vi "IR_PARA_00.vi"(8 "Parâmetros":T3={"Verde Min "=0.0, "Verde  MAX"=4.0, "Vemelho Max"=0, "Azul Max"=0, "Amarelo Max"=0, "Chão Max"=0.0, "Branco Max EV3 Cor"=0.0, "Branco Min EV3 Cor"=0.0, "Preto Max EV3 Cor"=0.0, "Preto Min EV3 Cor"=0.0, "Tubo CM Max"=0.0, "Tubo CM Min"=0.0, "Dist Proxima"=0.0, "Graus Emp"=0, "Graus Aprox"=0, "Graus Afast"=0, "180dg"=170.0, "90dg"=80.0, "Vemelho Min"=0, "Azul  Min"=0, "Amarelo Min"=0, "Chão Min"=0.0}, 11 "NXT/EV3":T2) -> (3 "NXT/EV3 2":T2)   [LabVIEW 2016]
uses:
  <vilib>/NXT/LegoClasses/BrickReference/BrickReference.lvclass
  <vilib>/NXT/Subs/LVHSConnector.ctl
  <vilib>/NXT/Block Support/NXT_OutputPort.ctl
  <vilib>/NXT/Dual Mode Library/Sensors/EV3_Color_Reflect.vi
  <vilib>/NXT/NXTIO Xnodes/NXTIONodeSubVIs/NXTStopMotors.vi
  <vilib>/NXT/NXTIO Xnodes/AddressXNode/NXTIOAddress.xnode
  <vilib>/NXT/NXTIO Xnodes/NXTIOXNode/NXTIO.xnode
panel:
  out "x+1":i32
  in  "Numeric":i32
  in  "Parâmetros\n CHÃO":T1={"Branco HiTechnic"=17, "Preto HiTechnic"=0, "Verde HiTechnic"=6, "Vemelho HiTechnic"=0, "Azul HiTechnic"=0, "Amarelo HiTechnic"=0, "Chão EV3 Cor"=0.0, "Branco Max EV3 Cor"=0.0, "Branco Min EV3 Cor"=0.0, "Preto Max EV3 Cor"=0.0, "Preto Min EV3 Cor"=0.0, "Tubo CM Max"=0.0, "Tubo CM Min"=0.0, "Dist Proxima"=0.0, "Graus Emp"=0, "Graus Aprox"=0, "Graus Afast"=0, "180dg"=0.0, "90dg"=0.0}
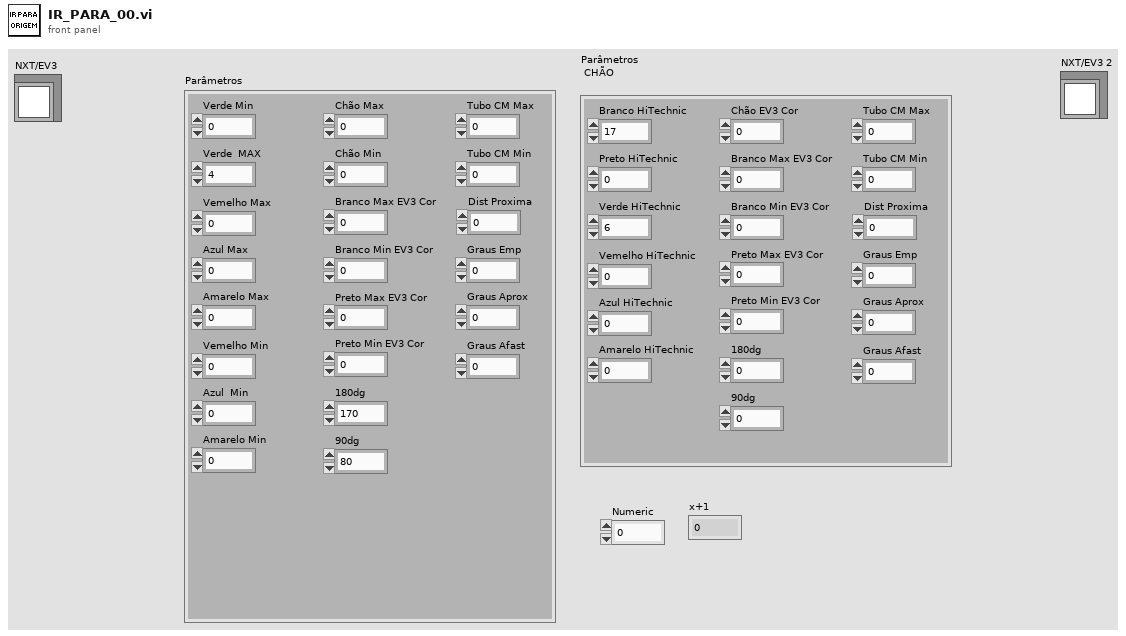
[diagram p1: front panel]
types:
  T1 = cluster{"Branco HiTechnic":i32, "Preto HiTechnic":i32, "Verde HiTechnic":i32, "Vemelho HiTechnic":i32, "Azul HiTechnic":i32, "Amarelo HiTechnic":i32, "Chão EV3 Cor":sgl, "Branco Max EV3 Cor":sgl, "Branco Min EV3 Cor":sgl, "Preto Max EV3 Cor":sgl, "Preto Min EV3 Cor":sgl, "Tubo CM Max":sgl, "Tubo CM Min":sgl, "Dist Proxima":dbl, "Graus Emp":i32, "Graus Aprox":i32, "Graus Afast":i32, "180dg":sgl, "90dg":sgl}
  T2 = typedef "LVHSConnector.ctl" = refnum<class "BrickReference.lvclass">
  T3 = cluster{"Verde Min ":dbl, "Verde  MAX":dbl, "Vemelho Max":i32, "Azul Max":i32, "Amarelo Max":i32, "Chão Max":sgl, "Branco Max EV3 Cor":sgl, "Branco Min EV3 Cor":sgl, "Preto Max EV3 Cor":sgl, "Preto Min EV3 Cor":sgl, "Tubo CM Max":sgl, "Tubo CM Min":sgl, "Dist Proxima":dbl, "Graus Emp":i32, "Graus Aprox":i32, "Graus Afast":i32, "180dg":sgl, "90dg":sgl, "Vemelho Min":i32, "Azul  Min":i32, "Amarelo Min":i32, "Chão Min":sgl}
  T4 = typedef "NXT_OutputPort.ctl" = u8
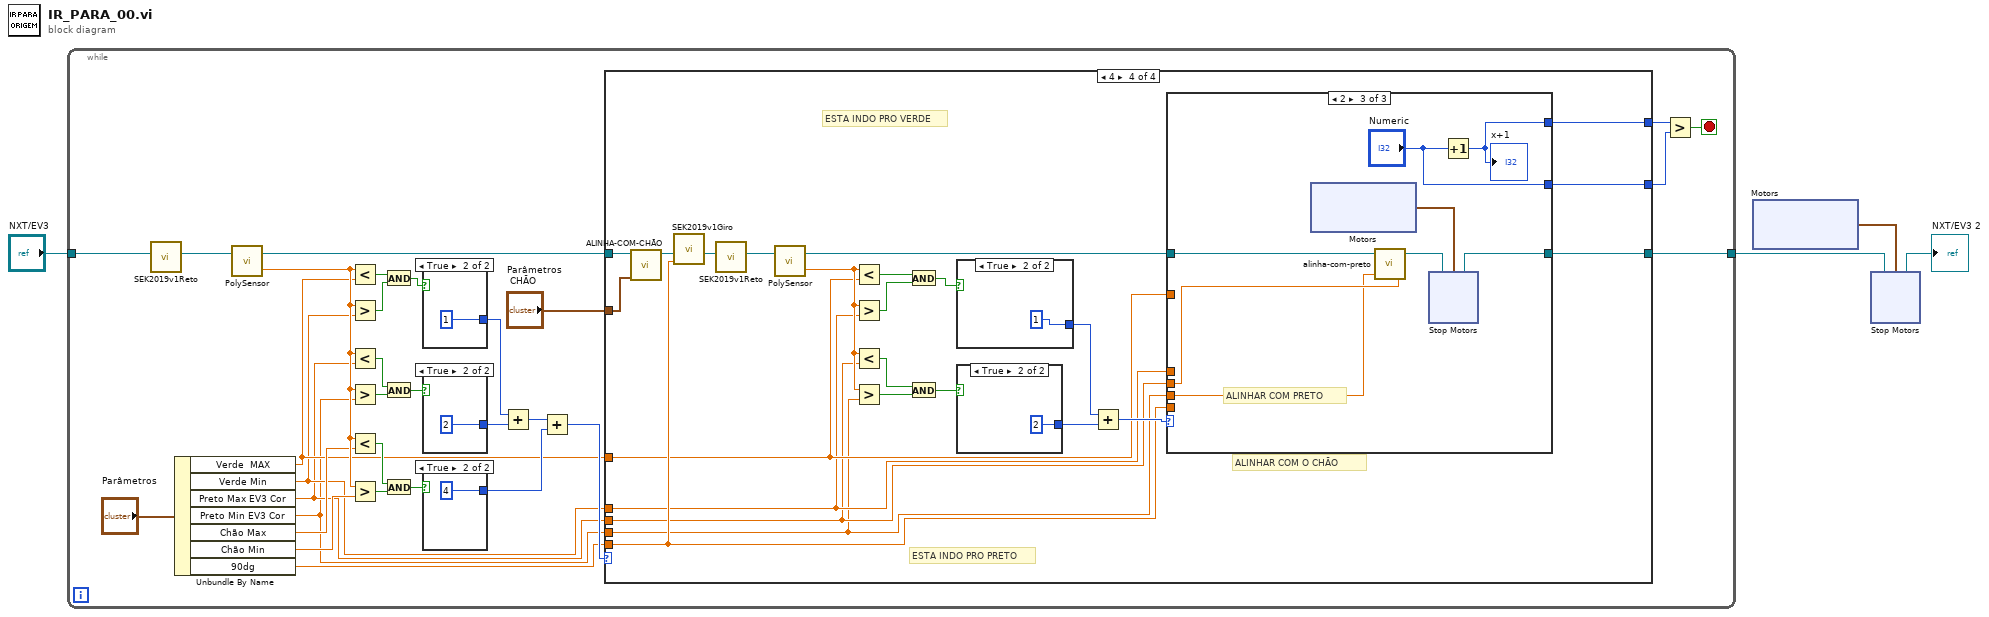
[diagram p0: block diagram]
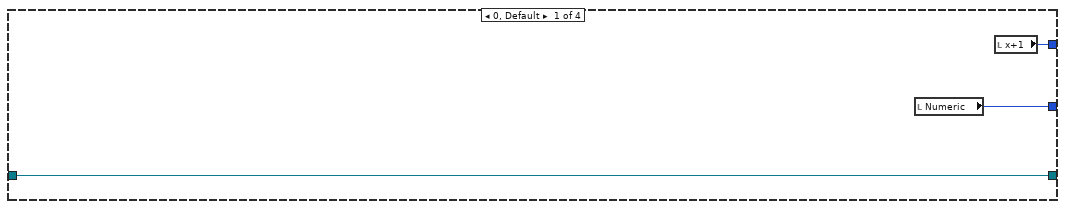
[diagram p2: hidden frame]
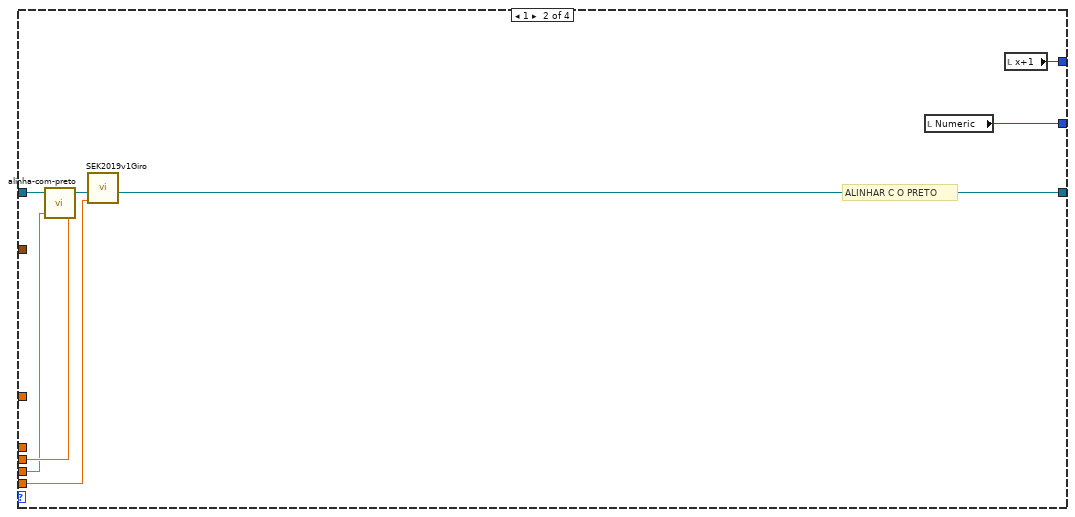
[diagram p3: hidden frame]
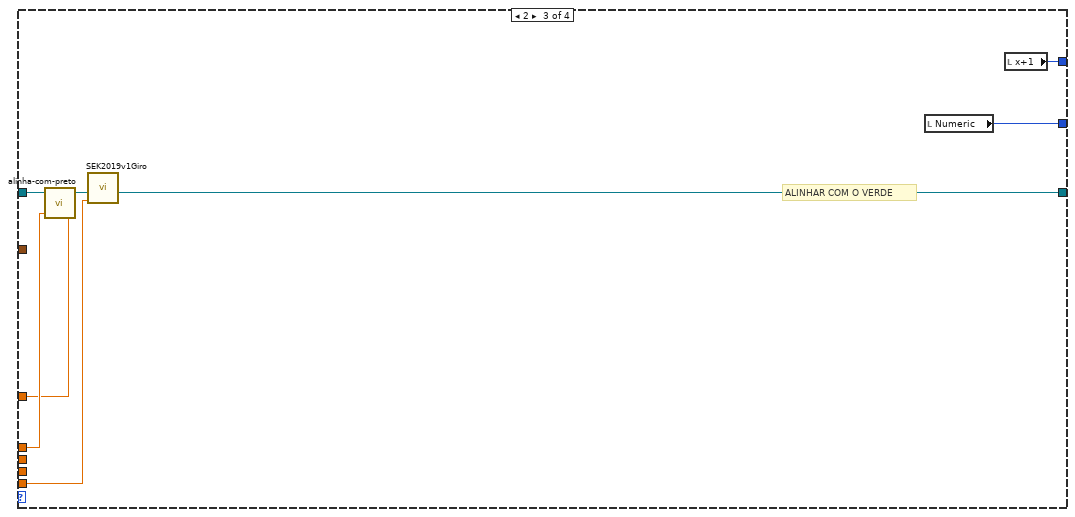
[diagram p4: hidden frame]
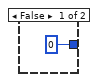
[diagram p5: hidden frame]
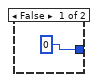
[diagram p6: hidden frame]
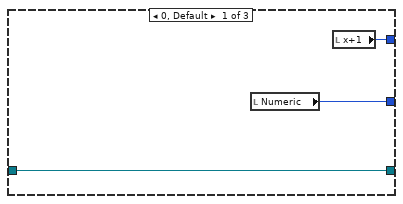
[diagram p7: hidden frame]
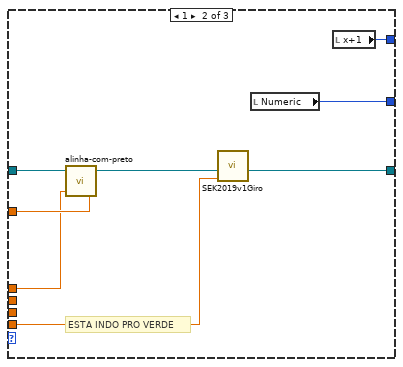
[diagram p8: hidden frame]
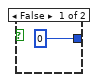
[diagram p9: hidden frame]
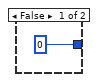
[diagram p10: hidden frame]
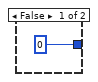
[diagram p11: hidden frame]
diagram:
  n1 = while {
    tunnel: "NXT/EV3" -> [w16]
    tunnel: [w9] -> w1
    stop <- w10 stop-if-true
    n2 = call "SEK2019v1Reto.vi"("NXT/EV3"=w16) -> ("NXT/EV3 2"=w15:T2)  [unwired: 10 in]
    n3 = Unbundle By Name("Parâmetros") -> ("Verde  MAX"=w8:dbl, "Verde Min"=w7:dbl, "Preto Max EV3 Cor"=w6:sgl, "Preto Min EV3 Cor"=w5:sgl, "Chão Max"=w28:sgl, "Chão Min"=w27:sgl, "90dg"=w14:sgl)
    n4 = call-poly <vilib>:"PolySensor.vi"("NXT/EV3"=w15) -> ("Scaled Value"=w29:sgl, "NXT/EV3"=w17:T2)  [unwired: 2 in]
    n5 = Less?(x=w29, y=w8) -> (x < y?=w21:bool)
    n6 = Greater?(x=w29, y=w7) -> (0:w22:bool)
    n7 = Less?(x=w29, y=w6) -> (x < y?=w24:bool)
    n8 = Greater?(x=w29, y=w5) -> (0:w23:bool)
    n9 = Less?(x=w29, y=w28) -> (x < y?=w26:bool)
    n10 = Greater?(x=w29, y=w27) -> (0:w25:bool)
    n11 = And(x=w21, y=w22) -> (x .and. y?=w20:bool)
    n12 = And(x=w24, y=w23) -> (x .and. y?=w19:bool)
    n13 = And(x=w26, y=w25) -> (x .and. y?=w18:bool)
    n14 = case shown="True" w20 {
      tunnel: [0 1] -> w34
      frame False {
      }
      frame True {
      }
    }
    n15 = case shown="True" w19 {
      tunnel: [0 2] -> w33
      frame False {
      }
      frame True {
      }
    }
    n16 = case shown="True" w18 {
      tunnel: [0 4] -> w32
      frame False {
      }
      frame True {
      }
    }
    n17 = Add(x=w34, y=w33) -> (x+y=w31:i32)
    n18 = Add(x=w31, y=w32) -> (x+y=w30:i32)
    n19 = case shown="4" w30 {
      tunnel: w8 -> [_ _ w53 w63]
      tunnel: w7 -> [_ _ w54 w62]
      tunnel: w6 -> [_ w46 _ w61]
      tunnel: w5 -> [_ w45 _ w60]
      tunnel: w17 -> [w38 w44 w52 w78]
      tunnel: [w38 w41 w50 w58] -> w9
      tunnel: w14 -> [_ w43 w49 w64]
      tunnel: "Parâmetros\n CHÃO" -> [_ _ _ w57]
      tunnel: [w37 w39 w48 w56] -> w12
      tunnel: [w36 w40 w47 w55] -> w11
      frame 0, Default {
        n20 = local read "Numeric"() -> (w37:i32)
        n21 = local read "x+1"() -> (w36:i32)
      }
      frame 1 {
        # "ALINHAR C O PRETO"
        n22 = call "alinha-com-preto.vi"("COR 2 Max EV3 Cor"=w46, "COR 2 Min EV3 Cor"=w45, "NXT/EV3"=w44) -> ("NXT/EV3 2"=w42:T2)  [unwired: 2 in]
        n23 = call "SEK2019v1Giro.vi"("ANGULO"=w43, "NXT/EV3"=w42) -> ("NXT/EV3 2"=w41:T2)  [unwired: 9 in]
        n24 = local read "Numeric"() -> (w39:i32)
        n25 = local read "x+1"() -> (w40:i32)
      }
      frame 2 {
        # "ALINHAR COM O VERDE"
        n26 = call "alinha-com-preto.vi"("COR 2 Max EV3 Cor"=w53, "COR 2 Min EV3 Cor"=w54, "NXT/EV3"=w52) -> ("NXT/EV3 2"=w51:T2)  [unwired: 2 in]
        n27 = call "SEK2019v1Giro.vi"("ANGULO"=w49, "NXT/EV3"=w51) -> ("NXT/EV3 2"=w50:T2)  [unwired: 9 in]
        n28 = local read "Numeric"() -> (w48:i32)
        n29 = local read "x+1"() -> (w47:i32)
      }
      frame 4 {
        # "ESTA INDO PRO VERDE"
        # "ESTA INDO PRO PRETO"
        # "ALINHAR COM O CHÃO"
        n30 = call "ALINHA-COM-CHÃO.vi"("Parâmetros"=w57, "NXT/EV3"=w78) -> ("NXT/EV3 2"=w77:T2)  [unwired: 9 in]
        n31 = call "SEK2019v1Giro.vi"("ANGULO"=w64, "NXT/EV3"=w77) -> ("NXT/EV3 2"=w76:T2)  [unwired: 9 in]
        n32 = call "SEK2019v1Reto.vi"("NXT/EV3"=w76) -> ("NXT/EV3 2"=w70:T2)  [unwired: 10 in]
        n33 = call-poly <vilib>:"PolySensor.vi"("NXT/EV3"=w70) -> ("Scaled Value"=w71:sgl, "NXT/EV3"=w59:T2)  [unwired: 2 in]
        n34 = Less?(x=w71, y=w63) -> (x < y?=w72:bool)
        n35 = Greater?(x=w71, y=w62) -> (0:w73:bool)
        n36 = Less?(x=w71, y=w61) -> (x < y?=w75:bool)
        n37 = Greater?(x=w71, y=w60) -> (0:w74:bool)
        n38 = And(x=w72, y=w73) -> (x .and. y?=w69:bool)
        n39 = And(x=w75, y=w74) -> (x .and. y?=w68:bool)
        n40 = case shown="True" w69 {
          tunnel: [0 1] -> w67
          frame False {
          }
          frame True {
          }
        }
        n41 = case shown="True" w68 {
          tunnel: [0 2] -> w66
          frame False {
          }
          frame True {
          }
        }
        n42 = Add(x=w67, y=w66) -> (x+y=w65:i32)
        n43 = case shown="2" w65 {
          tunnel: w64 -> [_ w92 _]
          tunnel: w63 -> [_ w91 _]
          tunnel: w62 -> [_ w90 _]
          tunnel: w61 -> [_ _ w101]
          tunnel: w60 -> [_ _ w100]
          tunnel: w59 -> [w85 w89 w99]
          tunnel: [w85 w88 w94] -> w58
          tunnel: [w83 w86 w96] -> w55
          tunnel: [w84 w87 "Numeric"] -> w56
          frame 0, Default {
            n44 = local read "Numeric"() -> (w84:i32)
            n45 = local read "x+1"() -> (w83:i32)
          }
          frame 1 {
            # "ESTA INDO PRO VERDE"
            n46 = call "alinha-com-preto.vi"("COR 2 Max EV3 Cor"=w91, "COR 2 Min EV3 Cor"=w90, "NXT/EV3"=w89) -> ("NXT/EV3 2"=w93:T2)  [unwired: 2 in]
            n47 = call "SEK2019v1Giro.vi"("ANGULO"=w92, "NXT/EV3"=w93) -> ("NXT/EV3 2"=w88:T2)  [unwired: 9 in]
            n48 = local read "Numeric"() -> (w87:i32)
            n49 = local read "x+1"() -> (w86:i32)
          }
          frame 2 {
            # "ALINHAR COM PRETO"
            n50 = xnode "Motors"() -> ("Motor"=w98:cluster{"Port":T4, "Port":T4})
            n51 = call "alinha-com-preto.vi"("COR 2 Max EV3 Cor"=w101, "COR 2 Min EV3 Cor"=w100, "NXT/EV3"=w99) -> ("NXT/EV3 2"=w97:T2)  [unwired: 2 in]
            n52 = xnode "Stop Motors"("Motors"=w98, "NXT/EV3"=w97) -> ("NXT/EV3"=w94:T2)
            n53 = Increment(x="Numeric") -> (x+1=w96:i32)
            "x+1" <- w96
          }
        }
      }
    }
    n54 = Greater?(x=w11, y=w12) -> (0:w10:bool)
  }
  n55 = xnode "Motors"() -> ("Motor"=w3:cluster{"Port":T4, "Port":T4})
  n56 = xnode "Stop Motors"("Motors"=w3, "NXT/EV3"=w1) -> ("NXT/EV3"=→"NXT/EV3 2":T2)
